vi "HFRR ADV v036.vi"() -> ()   [LabVIEW 2025] (continued)
                        n2404 = local read "NORMAL LOAD"() -> (w3460:dbl)
                        n2405 = Number To Fractional String(number=w3460, precision (6)=i16 2) -> (F-format string=w3461:string)  [unwired: 2 in]
                        n2406 = Concatenate Strings("Applied Load [grams] :" ("Content"), w3461) -> (w3463:string)
                        n2407 = local read "EVENT LOG"() -> (w3465:string)
                        n2408 = call "Event Log.vi"("Content"=w3463, "EVENT LOG"=w3465) -> ("EVENT LOG"=w3464:string)  [unwired: 8 in, 1 out]
                        n2409 = local write "EVENT LOG"(w3464) -> ()
                      }
                      frame #24 {
                        n2410 = Wait (ms)(milliseconds to wait=u32 50) -> ()  [unwired: 1 out]
                      }
                      frame #25 {
                        n2411 = local read "Set Strk"() -> (w3468:dbl)
                        n2412 = Number To Fractional String(number=w3468, precision (6)=i16 2) -> (F-format string=w3469:string)  [unwired: 2 in]
                        n2413 = Concatenate Strings("Set Stroke [mm] :" ("Content"), w3469) -> (w3471:string)
                        n2414 = local read "EVENT LOG"() -> (w3473:string)
                        n2415 = call "Event Log.vi"("Content"=w3471, "EVENT LOG"=w3473) -> ("EVENT LOG"=w3472:string)  [unwired: 8 in, 1 out]
                        n2416 = local write "EVENT LOG"(w3472) -> ()
                      }
                      frame #26 {
                        n2417 = Wait (ms)(milliseconds to wait=u32 50) -> ()  [unwired: 1 out]
                      }
                      frame #27 {
                        n2418 = local read "Set Temp"() -> (w3476:dbl)
                        n2419 = Number To Fractional String(number=w3476, precision (6)=i16 2) -> (F-format string=w3477:string)  [unwired: 2 in]
                        n2420 = Concatenate Strings("Set Temperature [deg C] :" ("Content"), w3477) -> (w3479:string)
                        n2421 = local read "EVENT LOG"() -> (w3481:string)
                        n2422 = call "Event Log.vi"("Content"=w3479, "EVENT LOG"=w3481) -> ("EVENT LOG"=w3480:string)  [unwired: 8 in, 1 out]
                        n2423 = local write "EVENT LOG"(w3480) -> ()
                      }
                      frame #28 {
                        n2424 = Wait (ms)(milliseconds to wait=u32 50) -> ()  [unwired: 1 out]
                      }
                      frame #29 {
                        n2425 = local read "Set Rh"() -> (w3484:dbl)
                        n2426 = Number To Fractional String(number=w3484, precision (6)=i16 2) -> (F-format string=w3485:string)  [unwired: 2 in]
                        n2427 = Concatenate Strings("Set Humidity [%RH] :" ("Content"), w3485) -> (w3487:string)
                        n2428 = local read "EVENT LOG"() -> (w3489:string)
                        n2429 = call "Event Log.vi"("Content"=w3487, "EVENT LOG"=w3489) -> ("EVENT LOG"=w3488:string)  [unwired: 8 in, 1 out]
                        n2430 = local write "EVENT LOG"(w3488) -> ()
                      }
                      frame #30 {
                        n2431 = Wait (ms)(milliseconds to wait=u32 50) -> ()  [unwired: 1 out]
                      }
                      frame #31 {
                        n2432 = local read "test time"() -> (w3492:dbl)
                        n2433 = Number To Fractional String(number=w3492, precision (6)=i16 1) -> (F-format string=w3493:string)  [unwired: 2 in]
                        n2434 = Concatenate Strings("Test Duration [mins] :" ("Content"), w3493) -> (w3495:string)
                        n2435 = local read "EVENT LOG"() -> (w3497:string)
                        n2436 = call "Event Log.vi"("Content"=w3495, "EVENT LOG"=w3497) -> ("EVENT LOG"=w3496:string)  [unwired: 8 in, 1 out]
                        n2437 = local write "EVENT LOG"(w3496) -> ()
                      }
                      frame #32 {
                        w3498 = dbl[] [] ("History Data")
                        w3499 = cluster{"y":dbl, dbl, "y":dbl}[] [] ("History Data")
                        w3500 = FALSE ("Visible")
                        n2438 = property on="Stroke ( mm )" class="WFChart (strict)"("History Data"=w3499) -> ()  [unwired: 2 in, 2 out]
                        n2439 = property on="Temperature ( Deg C )" class="WFChart (strict)"("History Data"=w3498) -> ()  [unwired: 2 in, 2 out]
                        n2440 = property on="Electrical Contact Resistance ( % )" class="WFChart (strict)"("History Data"=w3498) -> ()  [unwired: 2 in, 2 out]
                        n2441 = property on="Coefficient of Friction" class="WFChart (strict)"("History Data"=w3498) -> ()  [unwired: 2 in, 2 out]
                        n2442 = property on="Frictional Force ( N )" class="WFChart (strict)"("History Data"=w3498) -> ()  [unwired: 2 in, 2 out]
                        n2443 = property on="Coefficient of Friction" class="WFChart (strict)"("History Data"=w3498) -> ()  [unwired: 2 in, 2 out]
                        n2444 = property on="Frictional Force ( N )" class="WFChart (strict)"("History Data"=w3498) -> ()  [unwired: 2 in, 2 out]
                        n2445 = property on="Electrical Contact Resistance ( % )" class="WFChart (strict)"("History Data"=w3498) -> ()  [unwired: 2 in, 2 out]
                        n2446 = property on="Stroke ( mm )" class="WFChart (strict)"("History Data"=w3499) -> ()  [unwired: 2 in, 2 out]
                        n2447 = property on="Temperature ( Deg C )" class="WFChart (strict)"("History Data"=w3498) -> ()  [unwired: 2 in, 2 out]
                        n2448 = property on="Service Password Log" class="Str"("Visible"=w3500) -> ()  [unwired: 2 in, 2 out]
                        n2449 = property on="Password 3" class="Clust (strict)"("Visible"=w3500) -> ()  [unwired: 2 in, 2 out]
                      }
                    }
                    "TEST FILE NAM,E SAVED" <- TRUE ("TEST FILE NAM,E SAVED")
                  }
                }
              }
            }
          }
        }
        n2450 = local write "Test \nStatus"(w2889) -> ()
        n2451 = local write "Save"(w2889) -> ()
        n2452 = local read "Main Tab"() -> (w2883:T2)
        n2453 = case shown="True" w2886 {
          frame False {
            n2454 = local read "Rt 3"() -> (w2950:bool)
            n2455 = case shown="True" w2950 {
              frame False {
              }
              frame True {
                n2456 = local write "Rt 3"(FALSE ("Rt 3")) -> ()
              }
            }
            "Rt" <- TRUE ("Rt")
            "Rt 2" <- FALSE ("Rt")
          }
          frame True {
            n2457 = local read "Rt"() -> (w2956:bool)
            n2458 = local write "Rt 2"(TRUE ("Rt 2")) -> ()
            n2459 = case shown="True" w2956 {
              frame False {
              }
              frame True {
                n2460 = local write "Rt"(FALSE ("Rt")) -> ()
              }
            }
            "Rt 3" <- TRUE ("Rt 3")
          }
        }
        n2461 = case shown="\"Acquire\"" w2883 {
          tunnel: w2885 -> [_ w2985]
          frame Default {
            w2984 = 0.0 ("output")
            n2462 = local write "PID-out"(w2984) -> ()
            n2463 = local write "Frequency ( Hz )"(w2984) -> ()
            n2464 = local write "STROKE Initialize"(TRUE ("STROKE Initialize")) -> ()
          }
          frame "Acquire" {
            n2465 = stacked-sequence {
              frame #0 {
                n2466 = local read "Auto Start Test"() -> (w2987:bool)
                n2467 = case shown="True" w2987 {
                  tunnel: "RUN" -> [w3008 w3011]
                  tunnel: [w3008 w3010] -> w2988
                  frame False {
                  }
                  frame True {
                    n2468 = local read "Auto Start Temp"() -> (w3009:bool)
                    n2469 = Or(x=w3011, y=w3009) -> (x .or. y?=w3010:bool)
                  }
                }
                n2470 = local read "clk"() -> (w3007:dbl)
                n2471 = local read "Save"() -> (w3003:bool)
                n2472 = Equal?(x=w3007, y=0.0) -> (x = y?=w3004:bool)
                n2473 = And(x=w3004, y=w3003) -> (x .and. y?=w3005:bool)
                n2474 = Not(x="Engage") -> (.not. x?=w2994:bool)
                n2475 = case shown="False" w2988 {
                  tunnel: [0.0 w3034] -> w2990
                  frame False {
                    (unwired) TRUE ("Visible")
                    n2476 = local read "Auto Start Test"() -> (w3015:bool)
                    n2477 = local write "Start Time"(TRUE ("Start Time")) -> ()
                    n2478 = property on="Stroke 2" class="DigNum (strict)"("Visible"=FALSE) -> ()  [unwired: 2 in, 2 out]
                    n2479 = case shown="False" w3015 {
                      frame False {
                        n2480 = property on="Heater Button" class="Bool (strict)"("DisabledEnum"=T19."Enabled" ("Disabled")) -> ()  [unwired: 2 in, 2 out]
                        n2481 = property on="Humidity" class="Bool (strict)"("DisabledEnum"=T19."Enabled" ("Disabled")) -> ()  [unwired: 2 in, 2 out]
                      }
                      frame True {
                      }
                    }
                    n2482 = case shown="False" "TestCompFlg" {
                      frame False {
                        n2483 = local read "StartFlg"() -> (w3023:bool)
                        n2484 = case shown="True" w3023 {
                          frame False {
                          }
                          frame True {
                            n2485 = stacked-sequence {
                              frame #0 {
                                n2486 = local read "EVENT LOG"() -> (w3027:string)
                                n2487 = call "Event Log.vi"("Content"="Test was interrupted", "EVENT LOG"=w3027) -> ("EVENT LOG"=w3028:string)  [unwired: 8 in, 1 out]
                                n2488 = local write "EVENT LOG"(w3028) -> ()
                                n2489 = property on="RUN" class="Bool (strict)"("Visible"=TRUE) -> ()  [unwired: 2 in, 2 out]
                                n2490 = property on="Auto Start Test" class="Bool (strict)"("Visible"=TRUE) -> ()  [unwired: 2 in, 2 out]
                              }
                              frame #1 {
                                w3030 = FALSE ("StartFlg")
                                n2491 = property on="Heater Button" class="Bool (strict)"("Val(Sgnl)"=FALSE ("Value (Signaling)")) -> ()  [unwired: 2 in, 2 out]
                                n2492 = local write "Heater Button"(w3030) -> ()
                                n2493 = local write "StartFlg"(w3030) -> ()
                                n2494 = local write "Humidity"(w3030) -> ()
                              }
                              frame #2 {
                                n2495 = local write "Due Write"("VC;0" ("Command")) -> ()
                              }
                              frame #3 {
                                n2496 = Wait (ms)(milliseconds to wait=u32 1500) -> ()  [unwired: 1 out]
                              }
                              frame #4 {
                                n2497 = local write "Due Write"("HE;0" ("Command")) -> ()
                              }
                            }
                          }
                        }
                      }
                      frame True {
                      }
                    }
                    n2498 = local write "String 14"("Test will autostart once parameters reach the set value." ("String 14")) -> ()
                  }
                  frame True {
                    (unwired) FALSE ("Visible")
                    n2499 = property on="Stroke 2" class="DigNum (strict)"("Visible"=TRUE) -> ()  [unwired: 2 in, 2 out]
                    n2500 = property on="STOP 2" class="Bool (strict)"("Disabled"=u8 2) -> ()  [unwired: 2 in, 2 out]
                    n2501 = local write "String 14"(" Running....." ("String 14")) -> ()
                    n2502 = property on="Heater Button" class="Bool (strict)"("DisabledEnum"=T19."Disabled and Grayed Out" ("Disabled")) -> ()  [unwired: 2 in, 2 out]
                    n2503 = property on="Humidity" class="Bool (strict)"("DisabledEnum"=T19."Disabled and Grayed Out" ("Disabled")) -> ()  [unwired: 2 in, 2 out]
                    n2504 = case shown="True" "Start Time" {
                      selector: "Start Time" -> [_ w3053]
                      frame False {
                      }
                      frame True {
                        n2505 = Not(x=w3053) -> (.not. x?=w3052:bool)
                        n2506 = local write "Start Time"(w3052) -> ()
                        n2507 = local read "EVENT LOG"() -> (w3054:string)
                        n2508 = call "Event Log.vi"("Content"="Test in progress", "EVENT LOG"=w3054) -> ("EVENT LOG"=w3056:string)  [unwired: 8 in, 1 out]
                        n2509 = local write "EVENT LOG"(w3056) -> ()
                      }
                    }
                    n2510 = disable-structure shown="Enabled" {
                      disable-tunnel: [w3045 w3051] -> w3034
                      frame Disabled {
                        n2511 = local read "Set Hz"() -> (w3048:dbl)
                        n2512 = call <vilib>:"Uniform White Noise Waveform.vi"() -> ("signal out"=w3047:waveform(dbl))  [unwired: 10 in, 1 out]
                        n2513 = Random Number (0-1)() -> (number: 0 to 1=w3044:dbl)
                        n2514 = Add(x=w3048, y=w3047) -> (x+y=w3046:waveform(dbl))
                        n2515 = Multiply(x=ext 0.01 ("y"), y=w3044) -> (x*y=w3042:ext)
                        n2516 = Multiply(x=w3046, y=w3042) -> (x*y=w3045:waveform(ext))
                      }
                      frame Enabled {
                        n2517 = call-poly <vilib>:"Random Number (Range).vi"("lower bound (0)"=49.89, "upper bound (100)"=50.8) -> ("number"=w3051:dbl)  [unwired: 9 in]
                      }
                    }
                    "StartFlg" <- TRUE ("StartFlg")
                  }
                }
                n2518 = case shown="True" w3005 {
                  frame False {
                  }
                  frame True {
                    n2519 = local write "clk"(10.0 ("clk")) -> ()
                    n2520 = Get Date/Time In Seconds() -> (seconds since 1Jan1904=w3059:timestamp)
                    n2521 = To Double Precision Float(number=w3059) -> (double precision float=w3057:dbl)
                    n2522 = local write "acq timer"(w3057) -> ()
                    n2523 = local write "act save time"(w3057) -> ()
                  }
                }
                n2524 = call "Elapsed Time"("Time Target (s)"="Countdown", "Reset"=w2994) -> ("Elapsed Time (s)"=w2999:dbl, "Time has Elapsed"=w2997:bool)  [unwired: 10 in, 6 out]
                "Countdown 2" <- w2999
                n2525 = Subtract(x=w2999, y=2.0) -> (x-y=w3002:dbl)
                n2526 = Less?(x=w3002, y="Countdown") -> (x < y?=w3000:bool)
                n2527 = And(x=w3000, y=w2997) -> (x .and. y?=w2996:bool)
                n2528 = case shown="True" w2996 {
                  frame False {
                  }
                  frame True {
                    (unwired) dbl[] [] ("History Data")
                    n2529 = local write "Engage"(FALSE ("Engage")) -> ()
                    n2530 = local write "RUN"(TRUE ("RUN")) -> ()
                    n2531 = local read "Humidity ( %RH )"() -> (→"Rh Before":dbl)
                  }
                }
                n2532 = local read "Test \nStatus"() -> (w2992:bool)
                n2533 = Select(t=w2990, s=w2992, f=0.0) -> (s? t:f=w2991:dbl)
                n2534 = local write "Frequency ( Hz )"(w2991) -> ()
              }
              frame #1 {
                w3082 = 1000000.0 ("x")
                # "HC;1/0\nST;VALUE"
                # "Elapsed time\ncof\nstroke\nAir temp\nTemp\nHumidity"
                # "acq timer\n\nact save time"
                # "convert to microseconds"
                n2535 = local read "COUNT"() -> (w3065:i32)
                n2536 = local read "Rate"() -> (w3078:dbl)
                n2537 = Divide(x=w3082, y=w3078) -> (x/y=w3083:dbl)
                n2538 = Greater Or Equal?(x=w3065, y=250) -> (x >= y?=w3064:bool)
                n2539 = Get Date/Time In Seconds() -> (seconds since 1Jan1904=w3085:timestamp)
                n2540 = case shown="True" w3064 {
                  frame False {
                    n2541 = local read "COUNT"() -> (w3086:i32)
                    n2542 = Increment(x=w3086) -> (x+1=w3087:i32)
                    n2543 = local write "COUNT"(w3087) -> ()
                  }
                  frame True {
                    n2544 = local write "COUNT"(0 ("COUNT")) -> ()
                  }
                }
                n2545 = local read "Samplingtime 2"() -> (w3063:dbl)
                n2546 = local read "act save time"() -> (w3080:dbl)
                n2547 = Divide(x=w3083, y=w3082) -> (x/y=w3081:dbl)
                n2548 = To Double Precision Float(number=w3085) -> (double precision float=w3074:dbl)
                n2549 = Add(x=w3080, y=w3063) -> (x+y=w3079:dbl)
                n2550 = local read "acq timer"() -> (w3084:dbl)
                n2551 = local read "COUNT"() -> (w3067:i32)
                n2552 = Greater Or Equal?(x=w3074, y=w3079) -> (x >= y?=w3062:bool)
                n2553 = Multiply(x=w3081, y=w3067) -> (x*y=w3073:dbl)
                n2554 = Subtract(x=w3074, y=w3084) -> (x-y=w3076:dbl)
                n2555 = local read "Save"() -> (w3077:bool)
                n2556 = Add(x=w3076, y=w3073) -> (x+y=w3060:dbl)
                "Elapsed time 3" <- w3060
                n2557 = And(x=w3062, y=w3077) -> (x .and. y?=w3075:bool)
                n2558 = Divide(x=w3060, y=60.0) -> (x/y=w3071:dbl)
                n2559 = local read "Test \nStatus"() -> (w3061:bool)
                n2560 = local read "clk"() -> (w3068:dbl)
                n2561 = Equal?(x=w3068, y=10.0) -> (x = y?=w3070:bool)
                n2562 = case shown="True" w3075 {
                  tunnel: w3074 -> [_ w3200]
                  tunnel: [FALSE ("Boolean 2") TRUE ("Boolean 2")] -> _
                  frame False {
                  }
                  frame True {
                    w3154 = ";" ("Substring")
                    # "Pid out/\nFreq response value"
                    n2563 = local write "act save time"(w3200) -> ()
                    n2564 = local read "FILE"() -> (w3148:string)
                    n2565 = call "file check.vi"("file name in"=w3148) -> ("error out"=w3151:errorcluster, "file name out"=w3146:string)  [unwired: 9 in]
                    n2566 = local read "LVDT STROKE"() -> (w3143:dbl)
                    n2567 = local read "Add up Stroke"() -> (w3141:dbl)
                    n2568 = call "FILE PATH CREATION.vi"("error in"=w3151, "FILE NAME :"=w3146) -> ("FILE OUT"=w3149:path)  [unwired: 8 in, 1 out]
                    n2569 = local read "STROKE Initialize"() -> (w3136:bool)
                    n2570 = Concatenate Strings(w3146, ".dgf" ("Substring")) -> (w3150:string)
                    n2571 = Subtract(x=w3143, y=w3141) -> (x-y=w3142:dbl)
                    n2572 = Absolute Value(x=w3142) -> (abs(x)=w3139:dbl)
                    n2573 = local read "FF 2"() -> (→"Frictional Force ( N )" →"Frictional Force ( N )":dbl)
                    n2574 = Build Path(base path=w3149, name or relative path=w3150) -> (appended path=w3145:path)
                    n2575 = flat-sequence {
                      tunnel: w3139 -> [w3205]
                      tunnel: [w3204] -> w3137
                      tunnel: w3136 -> [w3202]
                      tunnel: [w3207] -> w3138
                      tunnel: w3137 -> [w3207]
                      frame #0 {
                        n2576 = call <vilib>:"Mean PtByPt.vi"("x"=w3205, "sample length"="STROKE FILTER", "initialize"=w3202) -> ("mean"=w3204:dbl)  [unwired: 1 in, 1 out]
                      }
                      frame #1 {
                        "STROKE Initialize" <- FALSE ("STROKE Initialize")
                      }
                    }
                    n2577 = local read "COF 2"() -> (w3159:dbl)
                    "Coefficient of Friction" <- w3159
                    "COF 4" <- w3159
                    "Coefficient of Friction" <- w3159
                    n2578 = local read "TEMP"() -> (w3162:dbl)
                    "Temperature ( Deg C )" <- w3162
                    n2579 = local read "Humidity ( %RH )"() -> (w3161:dbl)
                    n2580 = local read "Frequency ( Hz )"() -> (w3168:dbl)
                    n2581 = local read "LVDT STROKE DISPLAY"() -> (w3140:dbl)
                    n2582 = local read "Elapsed time"() -> (w3193:dbl)
                    n2583 = local read "AIR TEMP"() -> (w3166:dbl)
                    n2584 = local read "PID-out"() -> (w3171:dbl)
                    n2585 = local write "Temperature ( Deg C )"(w3162) -> ()
                    n2586 = Number To Fractional String(number=w3140, width (-)=i16 9 ("precision (6)"), precision (6)=i16 6) -> (F-format string=w3186:string)  [unwired: 1 in]
                    n2587 = Number To Fractional String(number=w3166, width (-)=i16 9 ("precision (6)"), precision (6)=i16 3) -> (F-format string=w3185:string)  [unwired: 1 in]
                    n2588 = Number To Fractional String(number=w3162, width (-)=i16 9 ("precision (6)"), precision (6)=i16 3) -> (F-format string=w3182:string)  [unwired: 1 in]
                    n2589 = Number To Fractional String(number=w3161, width (-)=i16 9 ("precision (6)"), precision (6)=i16 3) -> (F-format string=w3179:string)  [unwired: 1 in]
                    n2590 = Number To Fractional String(number=0.0, width (-)=i16 9 ("precision (6)"), precision (6)=i16 3) -> (F-format string=w3176:string)  [unwired: 1 in]
                    n2591 = Number To Fractional String(number=w3171, width (-)=i16 9 ("precision (6)"), precision (6)=i16 3) -> (F-format string=w3172:string)  [unwired: 1 in]
                    n2592 = Number To Fractional String(number=w3168, width (-)=i16 9 ("precision (6)"), precision (6)=i16 3) -> (F-format string=w3167:string)  [unwired: 1 in]
                    n2593 = Number To Fractional String(number=w3159, width (-)=i16 9 ("precision (6)"), precision (6)=i16 6) -> (F-format string=w3194:string)  [unwired: 1 in]
                    n2594 = Number To Fractional String(number=w3193, width (-)=i16 14 ("precision (6)"), precision (6)=i16 3) -> (F-format string=w3195:string)  [unwired: 1 in]
                    n2595 = Bundle("y"=1.02, "LVDT STROKE DISPLAY"=w3140, "y"=0.98) -> (w3160:T31)  [unwired: 1 in]
                    n2596 = Number To Fractional String(number="Ambient Humidity :", width (-)=i16 9 ("precision (6)"), precision (6)=i16 6) -> (F-format string=w3152:string)  [unwired: 1 in]
                    n2597 = local read "RUN"() -> (w3158:bool)
                    n2598 = case shown="True" w3158 {
                      tunnel: w3160 -> [_ w3211]
                      tunnel: w3140 -> [_ w3210]
                      tunnel: w3140 -> [_ w3208]
                      tunnel: w3140 -> [_ w3209]
                      frame False {
                      }
                      frame True {
                        "Stroke ( mm )" <- w3211
                        "Stroke ( mm )" <- w3211
                        "Stroke 4" <- w3210
                        "Stroke 3" <- w3208
                        "Stroke 2" <- w3209
                        "measured_stroke" <- w3208
                      }
                    }
                    n2599 = Concatenate Strings(w3195, w3154, w3194, w3154, w3186, w3154, w3185, w3154, w3182, w3154, w3179, w3154, w3176, w3154, w3172, w3154, w3167, w3154, w3152, "\r") -> (w3192:string)
                    n2600 = call <vilib>:"Write Characters To File.vi"("append to file? (new file:F)"=TRUE, "character string"=w3192, "file path (dialog if empty)"=w3145) -> ()  [unwired: 2 in, 1 out]
                    "refresh flag" <- TRUE ("refresh flag")
                    "LVDT STROKE Actual" <- w3138
                  }
                }
                n2601 = case shown="True" w3061 {
                  tunnel: w3071 -> [_ w3097]
                  tunnel: w3076 -> [_ w3107]
                  tunnel: [0.0 w3103] -> _
                  tunnel: w3070 -> [_ w3102]
                  tunnel: [0.0 w3101] -> _
                  tunnel: w3060 -> [_ w3101]
                  tunnel: w3074 -> [w3090 _]
                  frame False {
                    n2602 = local write "acq timer"(w3090) -> ()
                    n2603 = local write "Test Duration Status"(0.0 ("Test Duration Status")) -> ()
                  }
                  frame True {
                    n2604 = local read "Set Hz"() -> (w3104:dbl)
                    n2605 = local write "Elapsed time"(w3097) -> ()
                    n2606 = local read "test time"() -> (w3096:dbl)
                    n2607 = Multiply(x=w3107, y=w3104) -> (x*y=w3106:dbl)
                    n2608 = case shown="False" w3102 {
                      tunnel: w3106 -> [w3108 _]
                      tunnel: [w3108 1.0] -> w3103
                      frame False {
                        n2609 = local write "Cycles elapsed"(w3108) -> ()
                      }
                      frame True {
                      }
                    }
                    n2610 = Greater?(x=w3097, y=w3096) -> (0:w3105:bool)
                    n2611 = Subtract(x=w3096, y=w3097) -> (x-y=w3095:dbl)
                    n2612 = Multiply(x=w3095, y=60.0) -> (x*y=w3094:dbl)
                    n2613 = local write "Time Remaining"(w3094) -> ()
                    n2614 = local write "Remaining Time"(w3094) -> ()
                    n2615 = case shown="True" w3105 {
                      frame False {
                      }
                      frame True {
                        n2616 = stacked-sequence {
                          frame #0 {
                            w3113 = T19."Enabled" ("Disabled")
                            w3112 = FALSE ("TEST FILE NAM,E SAVED")
                            w3114 = "" ("FILE")
                            w3115 = TRUE ("Visible")
                            n2617 = local write "Humidity"(FALSE ("Humidity")) -> ()
                            n2618 = local write "RUN"(FALSE ("OK Button 2")) -> ()
                            n2619 = local write "Heater Button"(FALSE ("Heater Button")) -> ()
                            n2620 = local write "Auto Start Test"(FALSE ("Auto Start Test")) -> ()
                            n2621 = local write "TestCompFlg"(TRUE ("StpFlg")) -> ()
                            n2622 = local read "Humidity ( %RH )"() -> (→"Rh After":dbl)
                            n2623 = property on="STOP 2" class="Bool (strict)"("Disabled"=u8 0) -> ()  [unwired: 2 in, 2 out]
                            n2624 = local read "EVENT LOG"() -> (w3120:string)
                            n2625 = call "Event Log.vi"("Content"="Test Completed", "EVENT LOG"=w3120) -> ("EVENT LOG"=w3119:string)  [unwired: 8 in, 1 out]
                            n2626 = property on="RUN" class="Bool (strict)"("Visible"=w3115) -> ()  [unwired: 2 in, 2 out]
                            n2627 = property on="Auto Start Test" class="Bool (strict)"("Visible"=w3115) -> ()  [unwired: 2 in, 2 out]
                            n2628 = local write "Batch Ref Num :"(w3114) -> ()
                            n2629 = local write "FILE"(w3114) -> ()
                            n2630 = local write "EVENT LOG"(w3119) -> ()
                            n2631 = local write "TEST FILE NAM,E SAVED"(w3112) -> ()
                            n2632 = local write "Fuel Discription :"(w3114) -> ()
                            n2633 = local write "START TEMP"(w3112) -> ()
                            n2634 = local write "Remarks :"(w3114) -> ()
                            n2635 = local write "Main Dashboard Buttons"(T1."Imaging" ("Main Dashboard Buttons")) -> ()
                            n2636 = local write "Main Tab"(T2."Adv Scar" ("Main Tab")) -> ()
                            n2637 = property on="FRICVALZ 2" class="Bool (strict)"("DisabledEnum"=w3113) -> ()  [unwired: 2 in, 2 out]
                            n2638 = property on="FRICVALZ 3" class="Bool (strict)"("DisabledEnum"=w3113) -> ()  [unwired: 2 in, 2 out]
                            n2639 = property on="FRICVALZ 4" class="Bool (strict)"("DisabledEnum"=w3113) -> ()  [unwired: 2 in, 2 out]
                          }
                          frame #1 {
                            n2640 = Wait (ms)(milliseconds to wait=u32 1500) -> ()  [unwired: 1 out]
                          }
                          frame #2 {
                            n2641 = local write "Due Write"("VC;0") -> ()
                          }
                          frame #3 {
                            n2642 = Wait (ms)(milliseconds to wait=u32 1500) -> ()  [unwired: 1 out]
                          }
                          frame #4 {
                            n2643 = local write "Due Write"("VC;0") -> ()
                          }
                          frame #5 {
                            n2644 = Wait (ms)(milliseconds to wait=u32 1500) -> ()  [unwired: 1 out]
                          }
                          frame #6 {
                            n2645 = local write "Due Write"("ST;0") -> ()
                          }
                          frame #7 {
                            n2646 = local write "measured_stroke"(0.0 ("measured_stroke")) -> ()
                            n2647 = Wait (ms)(milliseconds to wait=u32 1500) -> ()  [unwired: 1 out]
                          }
                          frame #8 {
                            n2648 = local write "Due Write"("HE;0") -> ()
                          }
                        }
                      }
                    }
                    n2649 = Divide(x=w3097, y=w3096) -> (x/y=w3100:dbl)
                    n2650 = Multiply(x=w3100, y=100.0) -> (x*y=w3098:dbl)
                    n2651 = local write "Test Duration Status"(w3098) -> ()
                  }
                }
              }
              frame #2 {
                n2652 = case shown="True" "Heater Button" {
                  tunnel: [0.0 ("output") w3234] -> w3212
                  frame False {
                    w3215 = TRUE ("tmpchk")
                    n2653 = local read "TEMP"() -> (w3216:dbl)
                    n2654 = local write "Temp ini"(w3216) -> ()
                    n2655 = local write "Reset 4"(w3215) -> ()
                    n2656 = local write "tmpchk"(w3215) -> ()
                    n2657 = local write "reinit"(TRUE ("reinit")) -> ()
                    n2658 = local write "manual temp log"(TRUE ("manual temp log")) -> ()
                  }
                  frame True {
                    # "Logic to turn off\nthe heater when \ntemp is not rising.\nTime - 60 sec\nDelta t- 5°c"
                    n2659 = local read "Temp ini"() -> (w3223:dbl)
                    n2660 = local read "Auto Start Test"() -> (w3219:bool)
                    n2661 = Less?(x=w3223, y=53.0) -> (x < y?=w3221:bool)
                    n2662 = case shown="False" w3219 {
                      frame False {
                        n2663 = local read "Set Temp"() -> (w3243:dbl)
                        n2664 = local read "TEMP"() -> (w3242:dbl)
                        n2665 = Subtract(x=w3243, y=w3242) -> (x-y=w3241:dbl)
                        n2666 = Absolute Value(x=w3241) -> (abs(x)=w3240:dbl)
                        n2667 = Less?(x=w3240, y=0.5) -> (x < y?=w3238:bool)
                        n2668 = case shown="True" w3238 {
                          tunnel: "manual temp log" -> [_ w3244]
                          frame False {
                          }
                          frame True {
                            n2669 = case shown="True" w3244 {
                              selector: w3244 -> [_ w3245]
                              frame False {
                              }
                              frame True {
                                # "#Event log"
                                n2670 = Not(x=w3245) -> (.not. x?=w3246:bool)
                                n2671 = local write "manual temp log"(w3246) -> ()
                                n2672 = local read "EVENT LOG"() -> (w3249:string)
                                n2673 = call "Event Log.vi"("Content"="Target Temperature reached", "EVENT LOG"=w3249) -> ("EVENT LOG"=w3248:string)  [unwired: 8 in, 1 out]
                                n2674 = local write "EVENT LOG"(w3248) -> ()
                              }
                            }
                          }
                        }
                      }
                      frame True {
                        n2675 = local write "manual temp log"(TRUE ("manual temp log")) -> ()
                      }
                    }
                    n2676 = And(x="tmpchk", y=w3221) -> (x .and. y?=w3224:bool)
                    n2677 = case shown="True" w3224 {
                      frame False {
                      }
                      frame True {
                        n2678 = call "Elapsed Time8"("Time Target (s)"=300.0, "Reset"="Reset 4") -> ("Time has Elapsed"=w3251:bool)  [unwired: 10 in, 7 out]
                        n2679 = flat-sequence {
                          tunnel: w3251 -> [_]
                          frame #0 {
                            n2680 = local write "Reset 4"(FALSE ("Reset 4")) -> ()
                          }
                        }
                        n2681 = case shown="True" w3251 {
                          frame False {
                          }
                          frame True {
                            n2682 = local read "Temp ini"() -> (w3258:dbl)
                            n2683 = Add(x=w3258, y=5.0) -> (x+y=w3256:dbl)
                            n2684 = local read "TEMP"() -> (w3259:dbl)
                            n2685 = Greater?(x=w3259, y=w3256) -> (0:w3257:bool)
                            n2686 = case shown="False" w3257 {
                              frame False {
                                n2687 = local write "Heater Button"(FALSE ("Heater Button")) -> ()
                              }
                              frame True {
                                n2688 = local write "tmpchk"(FALSE ("tmpchk")) -> ()
                              }
                            }
                          }
                        }
                      }
                    }
                    n2689 = local read "Set Temp"() -> (w3232:dbl)
                    n2690 = local read "TEMP"() -> (w3226:dbl)
                    n2691 = call-poly <vilib>:"PID.vi"("reinitialize? (F)"="reinit", "dt (s)"=-1.0, "process variable"=w3226, "setpoint"=w3232) -> ("output"=w3229:dbl)  [unwired: 6 in, 1 out]
                    n2692 = Subtract(x=w3232, y=w3226) -> (x-y=w3233:dbl)
                    n2693 = Add(x=w3232, y=0.5) -> (x+y=w3230:dbl)
                    n2694 = Greater Or Equal?(x=w3226, y=w3230) -> ()  [unwired: 1 out]
                    n2695 = Select(t=0.0, s=FALSE, f=w3229) -> (s? t:f=w3228:dbl)
                    "PID output" <- w3228
                    n2696 = flat-sequence {
                      tunnel: w3228 -> [w3262]
                      tunnel: [w3262] -> w3234
                      frame #0 {
                        n2697 = local write "reinit"(FALSE ("reinit")) -> ()
                      }
                    }
                    n2698 = Bundle(w3233, "output"=w3228, "TEMP"=w3226) -> ()  [unwired: 1 in, 1 out]
                  }
                }
                "PID-out" <- w3212
              }
              frame #3 {
                n2699 = local read "TEMP"() -> (w3264:dbl)
                n2700 = Greater Or Equal?(x=w3264, y="Set Temp 2") -> (x >= y?=w3269:bool)
                n2701 = case shown="True" w3269 {
                  tunnel: [FALSE TRUE] -> w3267
                  frame False {
                  }
                  frame True {
                  }
                }
                "Status 13" <- w3267
                n2702 = And(x=w3267, y="trip1 8") -> (x .and. y?=w3266:bool)
                n2703 = case shown="True" w3266 {
                  frame False {
                    n2704 = local write "Heater Trip Temp"(TRUE ("Heater Trip Temp")) -> ()
                  }
                  frame True {
                    w3272 = FALSE ("OK Button 2")
                    n2705 = case shown="True" "Heater Trip Temp" {
                      selector: "Heater Trip Temp" -> [_ w3274]
                      frame False {
                      }
                      frame True {
                        n2706 = Not(x=w3274) -> (.not. x?=w3273:bool)
                        n2707 = local read "EVENT LOG"() -> (w3277:string)
                        n2708 = local write "Heater Trip Temp"(w3273) -> ()
                        n2709 = call "Event Log.vi"("Content"="Heater Trip", "EVENT LOG"=w3277) -> ("EVENT LOG"=w3276:string)  [unwired: 8 in, 1 out]
                        n2710 = local write "EVENT LOG"(w3276) -> ()
                      }
                    }
                    n2711 = local write "RUN"(w3272) -> ()
                    n2712 = property on="Auto Start Test" class="Bool (strict)"("Value"=w3272) -> ()  [unwired: 2 in, 2 out]
                    n2713 = local write "Heater Button"(w3272) -> ()
                  }
                }
              }
            }
            n2714 = case shown="False" w2985 {
              frame False {
                n2715 = disable-structure shown="Disabled" {
                  frame Disabled {
                    n2716 = stacked-sequence {
                      frame #0 {
                        n2717 = local write "RUN"(FALSE ("OK Button 2")) -> ()
                      }
                      frame #1 {
                      }
                    }
                  }
                  frame Enabled {
                  }
                }
              }
              frame True {
              }
            }
          }
        }
        n2718 = local read "Reset Graph"() -> (w2882:bool)
        n2719 = case shown="True" w2882 {
          selector: w2882 -> [_ w2899]
          frame False {
          }
          frame True {
            w2913 = 0.0 ("X Scale.Range:Maximum")
            n2720 = Not(x=w2899) -> (.not. x?=w2898:bool)
            n2721 = local write "Reset Graph"(w2898) -> ()
            n2722 = property on="Electrical Contact Resistance ( % )" class="WFChart (strict)"("XScale.Maximum"=600.0 ("X Scale.Range:Maximum"), "XScale.Minimum"=0.0 ("X Scale.Range:Minimum"), "YScale.Maximum"=100.0 ("Y Scale.Range:Maximum"), "YScale.Minimum"=0.0 ("Y Scale.Range:Minimum")) -> ()  [unwired: 2 in, 2 out]
            n2723 = property on="Frictional Force ( N )" class="WFChart (strict)"("XScale.Maximum"=600.0 ("X Scale.Range:Maximum"), "XScale.Minimum"=0.0 ("X Scale.Range:Minimum"), "YScale.Maximum"=100.0 ("Y Scale.Range:Maximum"), "YScale.Minimum"=0.0 ("Y Scale.Range:Minimum")) -> ()  [unwired: 2 in, 2 out]
            n2724 = property on="Temperature ( Deg C )" class="WFChart (strict)"("XScale.Maximum"=600.0 ("X Scale.Range:Maximum"), "XScale.Minimum"=0.0 ("X Scale.Range:Minimum"), "YScale.Maximum"=100.0 ("Y Scale.Range:Maximum"), "YScale.Minimum"=0.0 ("Y Scale.Range:Minimum")) -> ()  [unwired: 2 in, 2 out]
            n2725 = property on="Stroke ( mm )" class="WFChart (strict)"("XScale.Maximum"=600.0 ("X Scale.Range:Maximum"), "XScale.Minimum"=0.0 ("X Scale.Range:Minimum"), "YScale.Maximum"=100.0 ("Y Scale.Range:Maximum"), "YScale.Minimum"=0.0 ("Y Scale.Range:Minimum")) -> ()  [unwired: 2 in, 2 out]
            n2726 = property on="Coefficient of Friction" class="WFChart (strict)"("XScale.Maximum"=600.0 ("X Scale.Range:Maximum"), "XScale.Minimum"=0.0 ("X Scale.Range:Minimum"), "YScale.Maximum"=100.0 ("Y Scale.Range:Maximum"), "YScale.Minimum"=0.0 ("Y Scale.Range:Minimum")) -> ()  [unwired: 2 in, 2 out]
            n2727 = property on="Electrical Contact Resistance ( % )" class="WFChart (strict)"("XScale.Minimum"=0.0 ("X Scale.Range:Minimum"), "XScale.Maximum"=600.0 ("X Scale.Range:Maximum"), "YScale.Minimum"=0.0 ("Y Scale.Range:Minimum"), "YScale.Maximum"=100.0 ("Y Scale.Range:Maximum")) -> ()  [unwired: 2 in, 2 out]
            n2728 = property on="Temperature ( Deg C )" class="WFChart (strict)"("XScale.Minimum"=0.0 ("X Scale.Range:Minimum"), "XScale.Maximum"=600.0 ("X Scale.Range:Maximum"), "YScale.Minimum"=0.0 ("Y Scale.Range:Minimum"), "YScale.Maximum"=100.0 ("Y Scale.Range:Maximum")) -> ()  [unwired: 2 in, 2 out]
            n2729 = property on="Coefficient of Friction" class="WFChart (strict)"("XScale.Minimum"=0.0 ("X Scale.Range:Minimum"), "XScale.Maximum"=600.0 ("X Scale.Range:Maximum"), "YScale.Maximum"=1.0 ("X Scale.Range:Minimum"), "YScale.Minimum"=0.0 ("X Scale.Range:Minimum")) -> ()  [unwired: 2 in, 2 out]
            n2730 = property on="Frictional Force ( N )" class="WFChart (strict)"("XScale.Maximum"=600.0 ("X Scale.Range:Maximum"), "XScale.Minimum"=w2913, "YScale.Maximum"=10.0 ("Y Scale.Range:Maximum"), "YScale.Minimum"=w2913) -> ()  [unwired: 2 in, 2 out]
            n2731 = property on="Stroke ( mm )" class="WFChart (strict)"("XScale.Maximum"=600.0 ("X Scale.Range:Maximum"), "XScale.Minimum"=0.0 ("X Scale.Range:Minimum"), "YScale.Maximum"=100.0 ("Y Scale.Range:Maximum"), "YScale.Minimum"=0.0 ("Y Scale.Range:Minimum")) -> ()  [unwired: 2 in, 2 out]
          }
        }
      }
      frame "Compare Files" {
        # "Elapsed time\ncof\nstroke\nAir temp\nTemp\nHumidity"
        n2732 = case shown="True" "RSTV1 2" {
          frame False {
          }
          frame True {
            n2733 = property on="Humidity ( %RH )" class="XYGraph (strict)"("Y Scale.Display Format:Precision"=u8 0 ("Y Scale.Format & Precision:Precision")) -> ()  [unwired: 2 in, 2 out]
            n2734 = property on="Humidity ( %RH )" class="XYGraph (strict)"("X Scale.Range:Minimum"=0.0, "X Scale.Range:Maximum"=75.0, "Y Scale.Range:Minimum"=48.0, "Y Scale.Range:Maximum"=58.0) -> ()  [unwired: 2 in, 2 out]
          }
        }
        n2735 = case shown="True" "RST CP 2" {
          frame False {
          }
          frame True {
            n2736 = property on="XY Graph 13" class="XYGraph (strict)"("Y Scale.Display Format:Precision"=u8 0 ("Y Scale.Format & Precision:Precision")) -> ()  [unwired: 2 in, 2 out]
            n2737 = property on="XY Graph 13" class="XYGraph (strict)"("X Scale.Range:Minimum"=0.0, "X Scale.Range:Maximum"=75.0, "Y Scale.Range:Minimum"=0.0, "Y Scale.Range:Maximum"=100.0) -> ()  [unwired: 2 in, 2 out]
          }
        }
        n2738 = case shown="True" "RST CP" {
          frame False {
          }
          frame True {
            n2739 = property on="Sample Temperature ( °C )" class="XYGraph (strict)"("Y Scale.Display Format:Precision"=u8 2 ("Y Scale.Format & Precision:Precision")) -> ()  [unwired: 2 in, 2 out]
            n2740 = property on="Sample Temperature ( °C )" class="XYGraph (strict)"("X Scale.Range:Minimum"=0.0, "X Scale.Range:Maximum"=75.0, "Y Scale.Range:Minimum"=58.0, "Y Scale.Range:Maximum"=62.0) -> ()  [unwired: 2 in, 2 out]
          }
        }
        n2741 = case shown="True" "RSTV1 3" {
          frame False {
          }
          frame True {
            n2742 = property on="Air Temperature  ( °C )" class="XYGraph (strict)"("Y Scale.Display Format:Precision"=u8 2 ("Y Scale.Format & Precision:Precision")) -> ()  [unwired: 2 in, 2 out]
            n2743 = property on="Air Temperature  ( °C )" class="XYGraph (strict)"("X Scale.Range:Minimum"=0.0 ("Y Scale.Range:Minimum"), "X Scale.Range:Maximum"=75.0 ("Y Scale.Range:Maximum"), "Y Scale.Range:Minimum"=20.0 ("X Scale.Range:Minimum"), "Y Scale.Range:Maximum"=26.0 ("X Scale.Range:Maximum")) -> ()  [unwired: 2 in, 2 out]
          }
        }
        n2744 = case shown="True" "RSTV1 4" {
          frame False {
          }
          frame True {
            n2745 = property on="Stroke ( mm )" class="XYGraph (strict)"("Y Scale.Display Format:Precision"=u8 2 ("Y Scale.Format & Precision:Precision")) -> ()  [unwired: 2 in, 2 out]
            n2746 = property on="Stroke ( mm )" class="XYGraph (strict)"("X Scale.Range:Minimum"=0.0 ("Y Scale.Range:Maximum"), "X Scale.Range:Maximum"=75.0 ("X Scale.Range:Minimum"), "Y Scale.Range:Minimum"=0.98, "Y Scale.Range:Maximum"=1.02) -> ()  [unwired: 2 in, 2 out]
          }
        }
        n2747 = case shown="True" "rstv2" {
          frame False {
          }
          frame True {
            n2748 = property on="Coefficient Of Friction" class="XYGraph (strict)"("Y Scale.Display Format:Precision"=u8 3 ("Y Scale.Format & Precision:Precision")) -> ()  [unwired: 2 in, 2 out]
            n2749 = property on="Coefficient Of Friction" class="XYGraph (strict)"("X Scale.Range:Minimum"=0.0 ("Y Scale.Range:Maximum"), "X Scale.Range:Maximum"=75.0, "Y Scale.Range:Minimum"=0.0, "Y Scale.Range:Maximum"=1.0 ("X Scale.Range:Minimum")) -> ()  [unwired: 2 in, 2 out]
          }
        }
        n2750 = case shown="True" "RST CP 3" {
          frame False {
          }
          frame True {
            n2751 = property on="Air Temp ( °C ) vs Humidity ( % RH )" class="XYGraph (strict)"("X Scale.Range:Minimum"=18.0, "X Scale.Range:Maximum"=28.0 ("X Scale.Range:Minimum"), "Y Scale.Range:Minimum"=30.0 ("X Scale.Range:Minimum"), "Y Scale.Range:Maximum"=70.0 ("X Scale.Range:Minimum")) -> ()  [unwired: 2 in, 2 out]
          }
        }
        n2752 = case shown="True" "OPEN 1" {
          frame False {
          }
          frame True {
            (unwired) 0  # existing file
            w3553 = "Choose a datalog file to open"  # prompt
            n2753 = local write "OPEN 1"(FALSE ("OPEN 1")) -> ()
            n2754 = String To Path(string="C:\\LAB-IQ\\Data\\") -> (path=w3538:path)
            n2755 = File Dialog(6:"*.dgf" ("pattern"), 7:w3553, 11:w3538) -> (0:w3536:errorcluster, 3:w3544:path)  [unwired: 4 in, 2 out]
            n2756 = Unbundle(w3536) -> ()  [unwired: 3 out]
            n2757 = Strip Path(path=w3544) -> (name=w3543:string)  [unwired: 1 out]
            n2758 = Path To String(path=w3544) -> (string=w3539:string)
            "string1" <- w3539
            n2759 = Match Pattern(string=w3543, regular expression=".dgf") -> (before substring=→"String Control":string)  [unwired: 1 in, 3 out]
            n2760 = Match Pattern(string=w3539, regular expression=".dgf" ("substring (\"\")")) -> (before substring=w3549:string)  [unwired: 1 in, 3 out]
            n2761 = Concatenate Strings(w3549, ".duf" ("Substring")) -> (w3545:string)
            n2762 = String To Path(string=w3545) -> (path=w3550:path)
            n2763 = call <vilib>:"Read Characters From File.vi"("file path (dialog if empty)"=w3550, "start of read offset (chars.:0)"=60 ("start of read offset (chars.: 0)")) -> ("character string"=→"String Control 2":string)  [unwired: 4 in, 3 out]
          }
        }
        n2764 = case shown="True" "OPEN 2" {
          frame False {
          }
          frame True {
            (unwired) 0  # existing file
            w3571 = "Choose a datalog file to open"  # prompt
            n2765 = local write "OPEN 2"(FALSE ("OPEN 1")) -> ()
            n2766 = String To Path(string="C:\\LAB-IQ\\Data\\") -> (path=w3556:path)
            n2767 = File Dialog(6:"*.dgf" ("pattern"), 7:w3571, 11:w3556) -> (0:w3554:errorcluster, 3:w3562:path)  [unwired: 4 in, 2 out]
            n2768 = Unbundle(w3554) -> ()  [unwired: 3 out]
            n2769 = Strip Path(path=w3562) -> (name=w3560:string)  [unwired: 1 out]
            n2770 = Path To String(path=w3562) -> (string=w3557:string)
            "string1 2" <- w3557
            n2771 = Match Pattern(string=w3560, regular expression=".dgf") -> (before substring=→"String Control 3":string)  [unwired: 1 in, 3 out]
            n2772 = Match Pattern(string=w3557, regular expression=".dgf" ("substring (\"\")")) -> (before substring=w3568:string)  [unwired: 1 in, 3 out]
            n2773 = Concatenate Strings(w3568, ".duf" ("Substring")) -> (w3565:string)
            n2774 = String To Path(string=w3565) -> (path=w3563:path)
            n2775 = call <vilib>:"Read Characters From File.vi"("file path (dialog if empty)"=w3563, "start of read offset (chars.:0)"=60 ("start of read offset (chars.: 0)")) -> ("character string"=→"String Control 4":string)  [unwired: 4 in, 3 out]
          }
        }
        n2776 = case shown="True" "OPEN 3" {
          frame False {
          }
          frame True {
            (unwired) 0  # existing file
            w3589 = "Choose a datalog file to open"  # prompt
            n2777 = local write "OPEN 3"(FALSE ("OPEN 1")) -> ()
            n2778 = String To Path(string="C:\\LAB-IQ\\Data\\") -> (path=w3574:path)
            n2779 = File Dialog(6:"*.dgf" ("pattern"), 7:w3589, 11:w3574) -> (0:w3572:errorcluster, 3:w3580:path)  [unwired: 4 in, 2 out]
            n2780 = Unbundle(w3572) -> ()  [unwired: 3 out]
            n2781 = Strip Path(path=w3580) -> (name=w3578:string)  [unwired: 1 out]
            n2782 = Path To String(path=w3580) -> (string=w3575:string)
            "string1 3" <- w3575
            n2783 = Match Pattern(string=w3578, regular expression=".dgf") -> (before substring=→"String Control 5":string)  [unwired: 1 in, 3 out]
            n2784 = Match Pattern(string=w3575, regular expression=".dgf" ("substring (\"\")")) -> (before substring=w3585:string)  [unwired: 1 in, 3 out]
            n2785 = Concatenate Strings(w3585, ".duf" ("Substring")) -> (w3582:string)
            n2786 = String To Path(string=w3582) -> (path=w3586:path)
            n2787 = call <vilib>:"Read Characters From File.vi"("file path (dialog if empty)"=w3586, "start of read offset (chars.:0)"=60 ("start of read offset (chars.: 0)")) -> ("character string"=→"String Control 6":string)  [unwired: 4 in, 3 out]
          }
        }
        n2788 = case shown="True" "OPEN 4" {
          frame False {
          }
          frame True {
            (unwired) 0  # existing file
            w3607 = "Choose a datalog file to open"  # prompt
            n2789 = local write "OPEN 4"(FALSE ("OPEN 1")) -> ()
            n2790 = String To Path(string="C:\\LAB-IQ\\Data\\") -> (path=w3592:path)
            n2791 = File Dialog(6:"*.dgf" ("pattern"), 7:w3607, 11:w3592) -> (0:w3590:errorcluster, 3:w3598:path)  [unwired: 4 in, 2 out]
            n2792 = Unbundle(w3590) -> ()  [unwired: 3 out]
            n2793 = Strip Path(path=w3598) -> (name=w3596:string)  [unwired: 1 out]
            n2794 = Path To String(path=w3598) -> (string=w3593:string)
            "string1 4" <- w3593
            n2795 = Match Pattern(string=w3596, regular expression=".dgf") -> (before substring=→"String Control 7":string)  [unwired: 1 in, 3 out]
            n2796 = Match Pattern(string=w3593, regular expression=".dgf" ("substring (\"\")")) -> (before substring=w3603:string)  [unwired: 1 in, 3 out]
            n2797 = Concatenate Strings(w3603, ".duf" ("Substring")) -> (w3600:string)
            n2798 = String To Path(string=w3600) -> (path=w3604:path)
            n2799 = call <vilib>:"Read Characters From File.vi"("file path (dialog if empty)"=w3604, "start of read offset (chars.:0)"=60 ("start of read offset (chars.: 0)")) -> ("character string"=→"String Control 8":string)  [unwired: 4 in, 3 out]
          }
        }
      }
      frame "About" {
        # "Elapsed time\ncof\nstroke\nmean pos\nTemp\nHumidity"
        n2800 = disable-structure shown="Disabled" {
          frame Disabled {
            n2801 = case shown="True" "Export" {
              frame False {
              }
              frame True {
                w3629 = "                                      " ("string")
                w3631 = "\r"
                (unwired) i16 6 ("width (-)")
                w3708 = "\r"
                w3640 = "\r"
                n2802 = local write "Export"(FALSE ("Export")) -> ()
                n2803 = local read "String 29"() -> (w3677:string)
                n2804 = local read "String 34"() -> (w3665:string)
                n2805 = local read "String 35"() -> (w3660:string)
                n2806 = local read "String 37"() -> (w3656:string)
                n2807 = local read "String 36"() -> (w3653:string)
                n2808 = local read "String 38"() -> (w3650:string)
                n2809 = local read "String 39"() -> (w3647:string)
                n2810 = Match Pattern(string=w3677, regular expression=".dwm") -> (before substring=w3673:string)  [unwired: 1 in, 3 out]
                "before substring" <- w3673
                n2811 = local read "S 38"() -> (w3668:string)
                n2812 = local read "S 39"() -> (w3661:string)
                n2813 = local read "Temperature before test 2"() -> (w3697:dbl)
                n2814 = local read "Temperature after test 2"() -> (w3702:dbl)
                n2815 = local read "Humidity before test 2"() -> (w3683:dbl)
                n2816 = local read "Humidity after test 2"() -> (w3698:dbl)
                n2817 = local read "MWSD 2"() -> (w3694:dbl)
                n2818 = local read "WS1.4 2"() -> (w3710:dbl)
                n2819 = local read "HCF 2"() -> (w3706:dbl)
                n2820 = local read "AVP 2"() -> (w3695:dbl)
                n2821 = Concatenate Strings("1," ("string"), w3668) -> (w3667:string)
                n2822 = Concatenate Strings("2," ("string"), w3665) -> (w3664:string)
                n2823 = Concatenate Strings("3," ("string"), w3661) -> (w3663:string)
                n2824 = Concatenate Strings("4," ("string"), w3660) -> (w3659:string)
                n2825 = Concatenate Strings("5," ("string"), w3656) -> (w3657:string)
                n2826 = Concatenate Strings("6," ("string"), w3653) -> (w3654:string)
                n2827 = Concatenate Strings("7," ("string"), w3650) -> (w3651:string)
                n2828 = Concatenate Strings("8," ("string"), w3647) -> (w3648:string)
                n2829 = local read "Sample ID"() -> (w3715:string)
                n2830 = case shown="\"xlx\"" "Select File Type" {
                  tunnel: w3673 -> [w3718 w3720 w3722]
                  tunnel: [w3716 w3721 w3723] -> w3672
                  frame "xlx" {
                    n2831 = Concatenate Strings(w3718, ".xls" ("string")) -> (w3716:string)
                  }
                  frame "csv" {
                    n2832 = Concatenate Strings(w3720, ".csv" ("string")) -> (w3721:string)
                  }
                  frame "txt" {
                    n2833 = Concatenate Strings(w3722, ".txt" ("string")) -> (w3723:string)
                  }
                }
                n2834 = local read "Test Date"() -> (w3714:string)
                n2835 = local read "String 45"() -> (w3628:string)
                n2836 = local read "String 31"() -> (w3713:string)
                n2837 = local read "String 32"() -> (w3712:string)
                n2838 = local read "TITTLE"() -> (w3636:string)
                n2839 = Number To Fractional String(number=w3683, width (-)=i16 6, precision (6)=i16 2) -> (F-format string=w3682:string)  [unwired: 1 in]
                n2840 = Number To Fractional String(number=w3697, width (-)=i16 6, precision (6)=i16 2) -> (F-format string=w3703:string)  [unwired: 1 in]
                n2841 = Number To Fractional String(number=w3698, width (-)=i16 6, precision (6)=i16 2) -> (F-format string=w3696:string)  [unwired: 1 in]
                n2842 = Number To Fractional String(number=w3702, width (-)=i16 6, precision (6)=i16 2) -> (F-format string=w3701:string)  [unwired: 1 in]
                n2843 = Number To Fractional String(number=w3694, width (-)=i16 6, precision (6)=i16 2) -> (F-format string=w3692:string)  [unwired: 1 in]
                n2844 = Number To Fractional String(number=w3695, width (-)=i16 6, precision (6)=i16 2) -> (F-format string=w3693:string)  [unwired: 1 in]
                n2845 = Number To Fractional String(number=w3706, width (-)=i16 6, precision (6)=i16 2) -> (F-format string=w3707:string)  [unwired: 1 in]
                n2846 = Number To Fractional String(number=w3710, precision (6)=i16 2) -> (F-format string=w3711:string)  [unwired: 2 in]
                n2847 = local read "s.NO"() -> (w3630:string)
                n2848 = Concatenate Strings("=" ("string"), w3636) -> (w3635:string)
                n2849 = Concatenate Strings("S.No," ("string"), "                                       Parameters" ("string")) -> (w3641:string)
                n2850 = Concatenate Strings(w3708, w3667, w3682, w3708, w3664, w3703, w3708, w3663, w3696, w3708, w3659, w3701, w3708, w3657, w3692, w3708, w3654, w3693, w3708, w3651, w3707, w3708, w3648, w3711) -> (w3670:string)
                n2851 = Concatenate Strings(w3640, "," ("string"), w3628, w3630, w3629, w3712, w3715, w3629, w3713, w3714, w3640) -> (w3638:string)
                n2852 = local read "Tested by"() -> (w3644:string)
                n2853 = local read "String 33"() -> (w3645:string)
                n2854 = Concatenate Strings("," ("string"), "                                                                             " ("string")) -> (w3633:string)
                n2855 = Concatenate Strings(w3635, w3631, w3638, w3631, w3641, w3670, w3631, w3633, w3645, w3644) -> (→"export":string)
                n2856 = String To Path(string=w3672) -> (path=w3679:path)
                n2857 = local read "export"() -> (w3674:string)
                n2858 = call <vilib>:"Write Characters To File.vi"("append to file? (new file:F)"=FALSE, "character string"=w3674, "file path (dialog if empty)"=w3679) -> ()  [unwired: 2 in, 1 out]
              }
            }
          }
          frame Enabled {
          }
        }
        n2859 = case shown="True" "OK Button 17" {
          frame False {
          }
          frame True {
            (unwired) 0  # existing file
            w3932 = "Choose a datalog file to open"  # prompt
            n2860 = local write "OK Button 17"(FALSE ("OK Button 17")) -> ()
            n2861 = local read "String"() -> (w3927:string)
            n2862 = String To Path(string=w3927) -> (path=w3928:path)
            n2863 = File Dialog(6:"*.duf" ("pattern"), 7:w3932, 11:w3928) -> (0:w3919:errorcluster, 3:w3938:path)  [unwired: 4 in, 2 out]
            n2864 = Unbundle(w3919) -> ()  [unwired: 3 out]
            n2865 = Open/Create/Replace File "Open File"(file path (use dialog)=w3938) -> (refnum out=w3930:refnum<file>)  [unwired: 5 in, 2 out]
            n2866 = Strip Path(path=w3938) -> (name=w3936:string)  [unwired: 1 out]
            n2867 = Path To String(path=w3938) -> (string=w3921:string)
            n2868 = while {
              tunnel: w3930 -> [w3942]
              i -> [w3939]
              stop <- w3940 continue-if-true
              (unwired) TRUE ("line mode (F)")
              n2869 = Read from Text File "Read File"(file (use dialog)=w3942) -> (text=w3941:string)  [unwired: 3 in, 3 out]
              n2870 = local write "Numeric 16"(w3939) -> ()
              n2871 = String Length(string=w3941) -> (length=w3944:i32)
              n2872 = Greater?(x=w3944, y=1) -> (0:w3940:bool)
            }
            n2873 = local write "String 29"(w3921) -> ()
            n2874 = Search and Replace String(input string=w3921, search string=".duf", replace string=".dgf" ("replace string (\"\")")) -> (result string=→"String Indicator 4":string)  [unwired: 5 in, 3 out]
            n2875 = Match Pattern(string=w3936, regular expression=".dwm") -> (before substring=w3920:string)  [unwired: 1 in, 3 out]
            "String Indicator" <- w3920
            n2876 = Match Pattern(string=w3921, regular expression=".dwm" ("substring (\"\")")) -> (before substring=w3922:string)  [unwired: 1 in, 3 out]
            "String Indicator 3" <- w3922
            n2877 = local write "TITTLE 2"(w3920) -> ()
            n2878 = String To Path(string=w3922) -> (path=w3929:path)
            "path" <- w3929
            n2879 = call <vilib>:"Read Characters From File.vi"("file path (dialog if empty)"=w3929, "start of read offset (chars.:0)"=60 ("start of read offset (chars.: 0)")) -> ("character string"=→"String Indicator 2":string)  [unwired: 4 in, 3 out]
          }
        }
        n2880 = call <vilib>:"Query Available Printers.vi"() -> ("system configured printers"=w3621:string[])  [unwired: 9 in, 2 out]
        "System Configured Printers 2" <- w3621
        n2881 = local read "OK Button 16"() -> (w3618:bool)
        n2882 = case shown="True" "OK Button 16" {
          frame False {
          }
          frame True {
            n2883 = stacked-sequence {
              frame #0 {
                n2884 = local read "Numeric 16"() -> (w3946:i32)
                n2885 = local write "Numeric 10"(w3946) -> ()
              }
              frame #1 {
                n2886 = local read "String 29"() -> (w3949:string)
                n2887 = String To Path(string=w3949) -> (path=w3948:path)
                n2888 = Open/Create/Replace File "Open File"(file path (use dialog)=w3948) -> (refnum out=w3950:refnum<file>)  [unwired: 5 in, 2 out]
                n2889 = for {
                  N: 16 -> [_]
                  tunnel: w3950 -> [w3957]
                  i -> [w3953]
                  (unwired) TRUE ("line mode (F)")
                  n2890 = Read from Text File "Read File"(file (use dialog)=w3957) -> (text=w3951:string)  [unwired: 3 in, 3 out]
                  n2891 = Match Pattern(string=w3951, regular expression="(") -> (after substring=w3956:string)  [unwired: 1 in, 3 out]
                  n2892 = Match Pattern(string=w3956, regular expression=")") -> (before substring=w3952:string)  [unwired: 1 in, 3 out]
                  n2893 = case shown="1" w3953 {
                    tunnel: w3952 -> [w3958 w3959 _ _ w3960 w3961 w3962 w3964 w3966 w3968 w3970 w3972 w3974 w3976 _]
